vi "LIN show Tags.vi"(4 "Choose Sequence":T2) -> (1 "LIN show Tags":T1(tab))   [LabVIEW 2018]
uses:
  LIN sequence for self SCU.ctl
  05.UserVI's/type defs/Inalfa LIN Tags.ctl
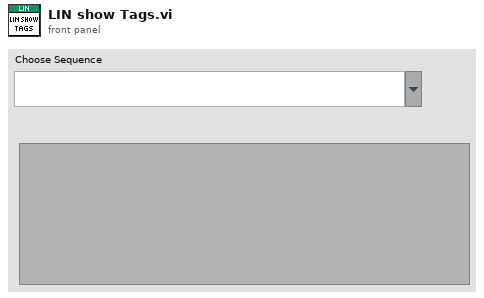
[diagram p1: front panel]
types:
  T1 = enum32{"Blank", "Cycles", "Read Cycles", "Software Level", "Hardware Level", "Calfile Level", "Tx", "Tx and Rx", "Go to position", "Check positions", "BYD Teach"}
  T2 = typedef "LIN sequence for self SCU.ctl" = string
  T3 = typedef "Inalfa LIN Tags.ctl" = enum32{"Blank", "Cycles", "Read Cycles", "Software Level", "Hardware Level", "Calfile Level", "Tx", "Tx and Rx", "Go to position", "Check positions", "BYD Teach"}
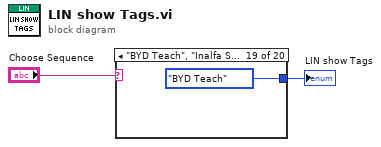
[diagram p0: block diagram]
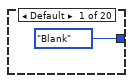
[diagram p2: hidden frame]
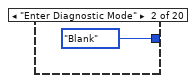
[diagram p3: hidden frame]
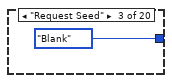
[diagram p4: hidden frame]
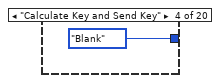
[diagram p5: hidden frame]
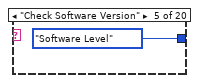
[diagram p6: hidden frame]
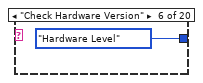
[diagram p7: hidden frame]
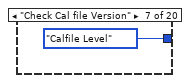
[diagram p8: hidden frame]
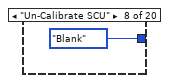
[diagram p9: hidden frame]
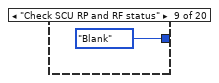
[diagram p10: hidden frame]
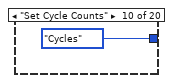
[diagram p11: hidden frame]
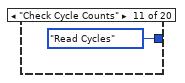
[diagram p12: hidden frame]
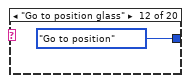
[diagram p13: hidden frame]
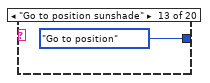
[diagram p14: hidden frame]
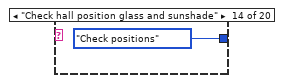
[diagram p15: hidden frame]
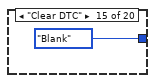
[diagram p16: hidden frame]
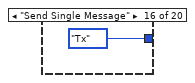
[diagram p17: hidden frame]
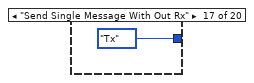
[diagram p18: hidden frame]
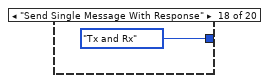
[diagram p19: hidden frame]
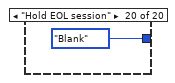
[diagram p20: hidden frame]
diagram:
  n1 = case shown="\"BYD Teach\", \"Inalfa SCU Teach\"" "Choose Sequence" {
    tunnel: [Inalfa_LIN_Tags."Blank" ("LIN show Tags 2") Inalfa_LIN_Tags."Blank" ("LIN show Tags 2") Inalfa_LIN_Tags."Blank" ("LIN show Tags 2") Inalfa_LIN_Tags."Blank" ("LIN show Tags 2") Inalfa_LIN_Tags."Software Level" ("LIN show Tags 2") Inalfa_LIN_Tags."Hardware Level" ("LIN show Tags 2") Inalfa_LIN_Tags."Calfile Level" ("LIN show Tags 2") Inalfa_LIN_Tags."Blank" ("LIN show Tags 2") Inalfa_LIN_Tags."Blank" ("LIN show Tags 2") Inalfa_LIN_Tags."Cycles" ("LIN show Tags 2") Inalfa_LIN_Tags."Read Cycles" ("LIN show Tags 2") Inalfa_LIN_Tags."Go to position" ("LIN show Tags 2") Inalfa_LIN_Tags."Go to position" ("LIN show Tags 2") Inalfa_LIN_Tags."Check positions" ("LIN show Tags 2") Inalfa_LIN_Tags."Blank" ("LIN show Tags 2") Inalfa_LIN_Tags."Tx" ("LIN show Tags 2") Inalfa_LIN_Tags."Tx" ("LIN show Tags 2") Inalfa_LIN_Tags."Tx and Rx" ("LIN show Tags 2") Inalfa_LIN_Tags."BYD Teach" ("LIN show Tags 2") Inalfa_LIN_Tags."Blank" ("LIN show Tags 2")] -> w1
    frame Default {
    }
    frame "Enter Diagnostic Mode" {
    }
    frame "Request Seed" {
    }
    frame "Calculate Key and Send Key" {
    }
    frame "Check Software Version" {
    }
    frame "Check Hardware Version" {
    }
    frame "Check Cal file Version" {
    }
    frame "Un-Calibrate SCU" {
    }
    frame "Check SCU RP and RF status" {
    }
    frame "Set Cycle Counts" {
    }
    frame "Check Cycle Counts" {
    }
    frame "Go to position glass" {
    }
    frame "Go to position sunshade" {
    }
    frame "Check hall position glass and sunshade" {
    }
    frame "Clear DTC" {
    }
    frame "Send Single Message" {
    }
    frame "Send Single Message With Out Rx" {
    }
    frame "Send Single Message With Response" {
    }
    frame "BYD Teach", "Inalfa SCU Teach" {
    }
    frame "Hold EOL session" {
    }
  }
  "LIN show Tags" <- w1
